vi "load tags from cvt1.vi"(10 "vi path":path, 11 "engine configuration in":refnum<class "engine configuration.lvclass">) -> (2 "load attempted":bool, 3 "engine configuration out":refnum<class "engine configuration.lvclass">)   [LabVIEW 2013, in "PL Framework Configuration Tool.lvlib" / "EngineTags.lvclass"]
uses:
  EngineTags.lvclass
  <vilib>/NI/Module Execution Interface/Engine Configuration/engine configuration.lvclass
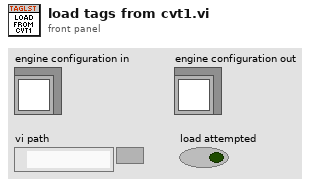
[diagram p1: front panel]
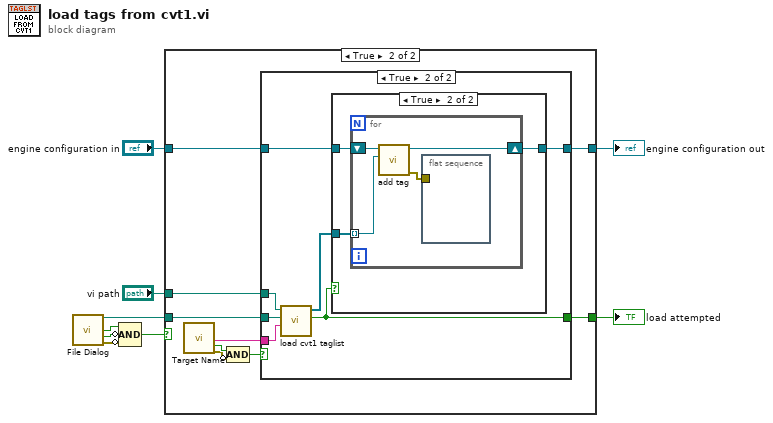
[diagram p0: block diagram]
diagram:
  n1 = call "File Dialog"() -> ("selected path"=w4:path, "exists"=w3:bool, "cancelled"=w2:bool, "error out"=w1:errorcluster)  [unwired: 12 in]
  n2 = Compound Arithmetic op=AND(w3, invert w2, invert w1) -> (w5:bool)
  n3 = case shown="True" w5 {
    tunnel: w4 -> [_ w19]
    tunnel: [_ w14] -> w9
    tunnel: "vi path" -> [_ w13]
    tunnel: [w10 w12] -> w7
    tunnel: "engine configuration in" -> [w10 w11]
    frame False {
    }
    frame True {
      n4 = call "Target Name"() -> ("Target Name"=w18:string, "OK"=w17:bool, "error out"=w16:errorcluster)  [unwired: 17 in]
      n5 = Compound Arithmetic op=AND(w17, invert w16) -> (w15:bool)
      n6 = case shown="True" w15 {
        tunnel: w19 -> [_ w26]
        tunnel: w18 -> [_ w25]
        tunnel: [_ w24] -> w14
        tunnel: w13 -> [_ w23]
        tunnel: [w20 w22] -> w12
        tunnel: w11 -> [w20 w21]
        frame False {
        }
        frame True {
          n7 = call "load cvt1 taglist.vi"("target name"=w25, "cfg file path"=w26, "vi path"=w23) -> ("ok?"=w24:bool, "tags"=w27:refnum<class "tag descriptor.lvclass">[])  [unwired: 7 in]
          n8 = case shown="True" w24 {
            tunnel: w27 -> [_ w29]
            tunnel: [w28 w31] -> w22
            tunnel: w21 -> [w28 w30]
            frame False {
            }
            frame True {
              n9 = for {
                shift-right: [w35] -> w31
                shift-left: w30 -> [w34]
                tunnel: w29 -> [w33] mode=indexing
                n10 = call <vilib>:"add tag.vi"("tag descriptor"=w33, "engine configuration in"=w34) -> ("error out"=w32:errorcluster, "engine configuration out"=w35:refnum<class "engine configuration.lvclass">)  [unwired: 8 in]
                n11 = flat-sequence {
                  tunnel: w32 -> [_]
                  frame #0 {
                  }
                }
              }
            }
          }
        }
      }
    }
  }
  "load attempted" <- w9
  "engine configuration out" <- w7
